vi "Keithley2100.contents.vi"   [LabVIEW 2014, in "Keithley2100.lvlib"]
doc: "This is the constructor of the Keithley2100 class."
uses:
  Keithley2100.lvlib
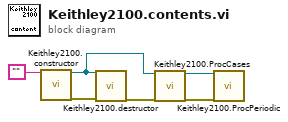
[diagram p0: block diagram]
diagram:
  n1 = call "Keithley2100.constructor.vi"("name"="") -> ("i ref out"=w6:refnum<vi>, "error out"=w4:errorcluster)  [unwired: 16 in, 1 out]
  n2 = call "Keithley2100.destructor.vi"("i ref in"=w6, "error in (no error)"=w4) -> ("error out"=w3:errorcluster)  [unwired: 17 in]
  n3 = call "Keithley2100.ProcCases.vi"("i ref in"=w6, "error in (no error)"=w3) -> ("i ref out"=w5:refnum<vi>, "error out"=w2:errorcluster)  [unwired: 15 in, 1 out]
  n4 = call "Keithley2100.ProcPeriodic.vi"("i ref in"=w5, "error in (no error)"=w2) -> ()  [unwired: 15 in, 3 out]
